vi "Data Global.vi"(7 "Write (F)":bool, 11 "Data IN":dbl) -> (3 "Data OUT":dbl)   [LabVIEW 2019]
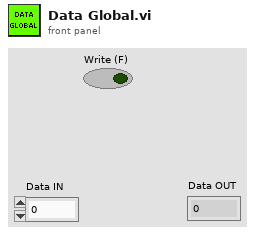
[diagram p1: front panel]
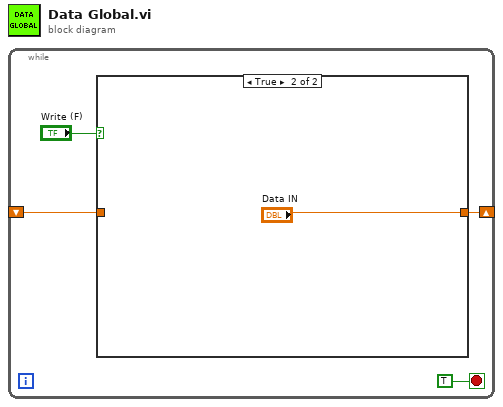
[diagram p0: block diagram]
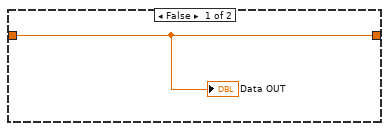
[diagram p2: hidden frame]
diagram:
  n1 = while {
    shift-right: [w2] -> _
    shift-left: _ -> [w1]
    stop <- TRUE stop-if-true
    n2 = case shown="True" "Write (F)" {
      tunnel: [w5 "Data IN"] -> w2
      tunnel: w1 -> [w5 _]
      frame False {
        "Data OUT" <- w5
      }
      frame True {
      }
    }
  }
